vi "_TangoReadStateImageAttribute.vi"(3 "error in":errorcluster, 4 "attribute name":string, 5 "device name":string) -> (0 "error out":errorcluster, 1 "setpoint":T1[][](array[typedef]), 2 "value":T1[][](array[typedef]))   [LabVIEW 2014, in "tango.lvlib"]
uses:
  tango.lvlib
  Common VIs/Typedefs/_TangoState_t.ctl
  Common VIs/Typedefs/_AttributeDataType_t.ctl
  Extractors/base/toStateImage.vi
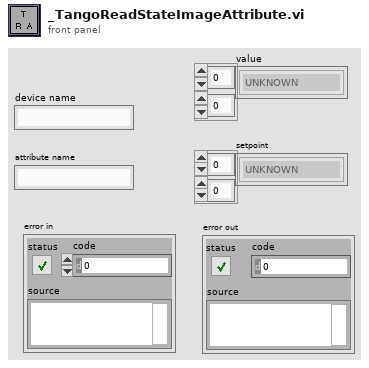
[diagram p1: front panel]
types:
  T1 = typedef "tango.lvlib/_TangoState_t.ctl" = enum32{"ON", "OFF", "CLOSE", "OPEN", "INSERT", "EXTRACT", "MOVING", "STANDBY", "FAULT", "INIT", "RUNNING", "ALARM", "DISABLE", "UNKNOWN"}
  T2 = typedef "tango.lvlib/_AttributeDataType_t.ctl" = enum16{"STATE_SCA", "STATE_SPE", "STATE_IMG", "STRING_SCA", "STRING_SPE", "STRING_IMG", "BOOL_SCA", "BOOL_SPE", "BOOL_IMG", "UCHAR_SCA", "UCHAR_SPE", "UCHAR_IMG", "SHORT_SCA", "SHORT_SPE", "SHORT_IMG", "USHORT_SCA", "USHORT_SPE", "USHORT_IMG", "LONG_SCA", "LONG_SPE", "LONG_IMG", "ULONG_SCA", "ULONG_SPE", "ULONG_IMG", "LONG64_SCA", "LONG64_SPE", "LONG64_IMG", "ULONG64_SCA", "ULONG64_SPE", "ULONG64_IMG", "FLOAT_SCA", "FLOAT_SPE", "FLOAT_IMG", "DOUBLE_SCA", "DOUBLE_SPE", "DOUBLE_IMG", "ENUM_SCA", "UNKNOWN_DATA_TYPE"}
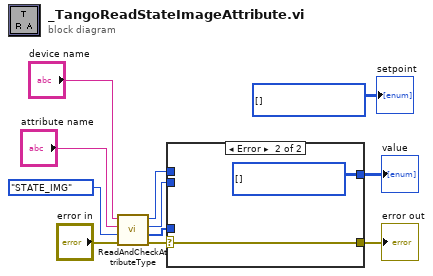
[diagram p0: block diagram]
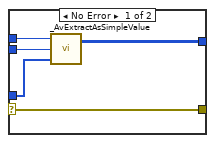
[diagram p2: hidden frame]
diagram:
  w5 = T1[][] [] items=["ON", "OFF", "CLOSE", "OPEN", "INSERT", "EXTRACT", "MOVING", "STANDBY", "FAULT", "INIT", "RUNNING", "ALARM", "DISABLE", "UNKNOWN"] ("setpoint")
  n1 = call "ReadAndCheckAttributeType.vi"("error in (no error)"="error in", "expected data type"=_AttributeDataType_t."STATE_IMG" ("Control"), "attribute name"="attribute name", "device name"="device name") -> ("error out"=w11:errorcluster, "value"=w8:u8[], "dim. y"=w9:i32, "dim. x"=w10:i32)  [unwired: 4 in]
  n2 = case shown="Error" w11 {
    selector: w11 -> [w12 w17]
    tunnel: w10 -> [w16 _]
    tunnel: w9 -> [w15 _]
    tunnel: w8 -> [w14 _]
    tunnel: [w12 w17] -> w6
    tunnel: [w13 w18] -> w4
    frame No Error {
      n3 = call-poly "_AvExtractAsSimpleValue.vi"("value_in"=w14, "dim_y"=w15, "dim_x"=w16) -> ("value_out"=w13:T1[][])  [unwired: 1 out]
    }
    frame Error {
      w18 = T1[][] [] items=["ON", "OFF", "CLOSE", "OPEN", "INSERT", "EXTRACT", "MOVING", "STANDBY", "FAULT", "INIT", "RUNNING", "ALARM", "DISABLE", "UNKNOWN"] ("value_out")
    }
  }
  "error out" <- w6
  "value" <- w4
  "setpoint" <- w5
